vi "set_V_value.vi"() -> ()   [LabVIEW 2017]
uses:
  types/motech_set_value_cluster.ctl
  types/channels_enum.ctl
panel:
  in  "motech_set_null":T1={"voltage"=0.0, "current"=0.0, "channel"=enum."1"}
  in  "current":dbl
  in  "negative_channel":T2=enum."1"
  in  "Numeric":dbl
  in  "positive_channel":T2=enum."1"
  in  "motech_set_active_value":T1={"voltage"=0.0, "current"=0.0, "channel"=enum."1"}
  in  "VISA resource name":refnum<visa-resource-name>
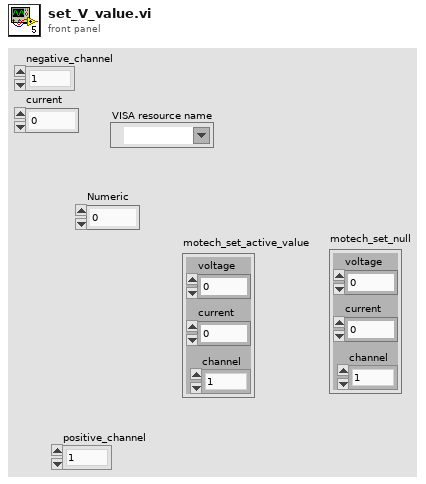
[diagram p1: front panel]
types:
  T1 = typedef "motech_set_value_cluster.ctl" = cluster{"voltage":dbl, "current":dbl, "channel":T2}
  T2 = typedef "channels_enum.ctl" = enum16{"0", "1", "2"}
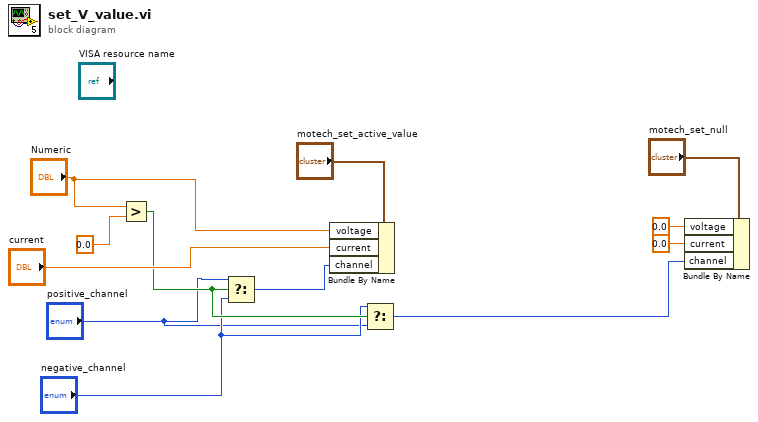
[diagram p0: block diagram]
diagram:
  n1 = Greater?(x="Numeric", y=0.0) -> (0:w4:bool)
  n2 = Select(t="positive_channel", s=w4, f="negative_channel") -> (s? t:f=w8:T2)
  n3 = Bundle By Name(cluster="motech_set_active_value", "voltage"="Numeric", "current"="current", "channel"=w8) -> ()  [unwired: 1 out]
  n4 = Select(t="negative_channel", s=w4, f="positive_channel") -> (s? t:f=w1:T2)
  n5 = Bundle By Name(cluster="motech_set_null", "voltage"=0.0, "current"=0.0, "channel"=w1) -> ()  [unwired: 1 out]
